vi "Panel Control State.vi"(8 "error in (no error)":errorcluster, 10 "Editable(True)":bool=TRUE, 11 "Panel Controls and VI Refnum":T1) -> (0 "error out":errorcluster, 3 "Panel Controls and VI Refnum out":T1)   [LabVIEW 2015, in "Panel Controller.lvclass"]
uses:
  Panel Controller.lvclass
  Panel Control/Panel Data/Type Definition/Panel Controls and VI Refnum.ctl
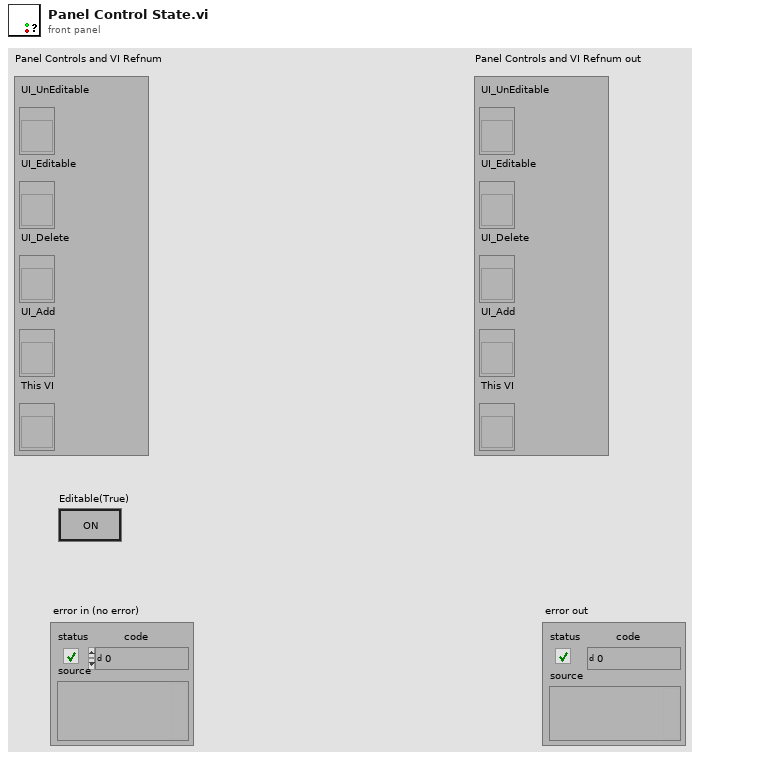
[diagram p1: front panel]
types:
  T1 = typedef "Panel Controller.lvclass/Panel Controls and VI Refnum.ctl" = cluster{"UI_UnEditable":refnum<vi>, "UI_Editable":refnum<vi>, "UI_Delete":refnum<vi>, "UI_Add":refnum<vi>, "This VI":refnum<vi>}
  T2 = enum8{"Enabled", "Disabled", "Disabled and Grayed Out"}
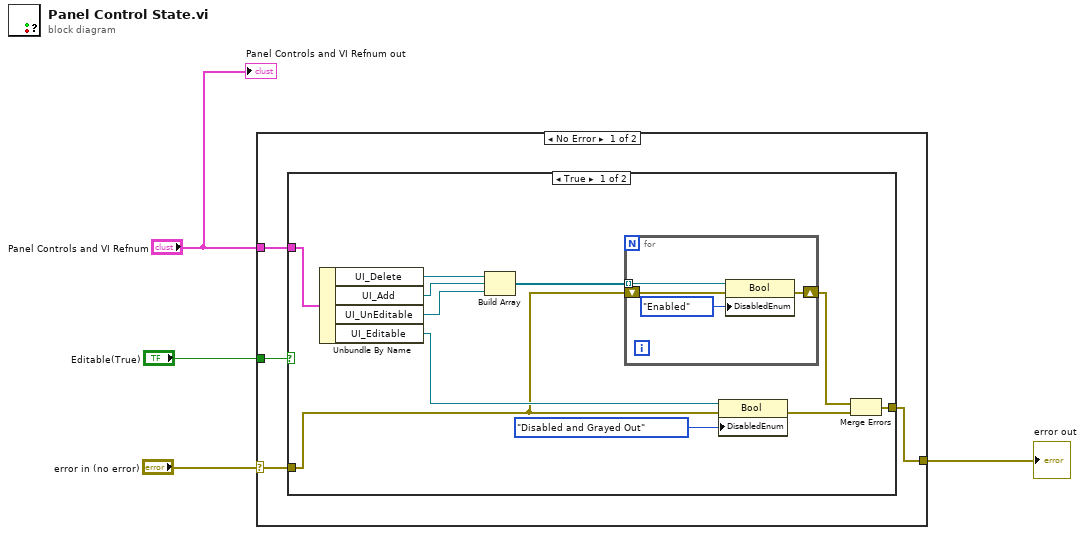
[diagram p0: block diagram]
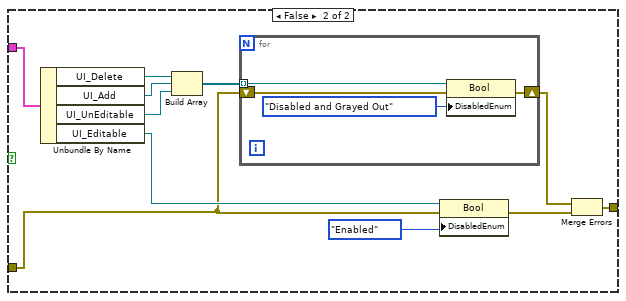
[diagram p2: hidden frame]
diagram:
  n1 = case shown="No Error" "error in (no error)" {
    selector: "error in (no error)" -> [w6 w39]
    tunnel: "Editable(True)" -> [w8 _]
    tunnel: "Panel Controls and VI Refnum" -> [w7 _]
    tunnel: [w5 w39] -> w1
    frame No Error {
      n2 = case shown="True" w8 {
        tunnel: w7 -> [w19 w34]
        tunnel: w6 -> [w12 w27]
        tunnel: [w9 w24] -> w5
        frame True {
          n3 = Unbundle By Name(w19) -> ("UI_Delete"=w18:refnum<vi>, "UI_Add"=w17:refnum<vi>, "UI_UnEditable"=w16:refnum<vi>, "UI_Editable"=w14:refnum<vi>)
          n4 = Build Array(w18, w17, w16) -> (w15:refnum<vi>[])
          n5 = for {
            tunnel: w15 -> [w23] mode=indexing
            shift-right: [w20] -> w11
            shift-left: w12 -> [w21]
            n6 = property class="Bool"(reference=w23, error in=w21, "DisabledEnum"=T2."Enabled" ("Disabled")) -> (error out=w20:errorcluster)  [unwired: 1 out]
          }
          n7 = property class="Bool"(reference=w14, error in=w12, "DisabledEnum"=T2."Disabled and Grayed Out" ("Disabled")) -> (error out=w10:errorcluster)  [unwired: 1 out]
          n8 = Merge Errors(w11, w10) -> (w9:errorcluster)
        }
        frame False {
          n9 = Unbundle By Name(w34) -> ("UI_Delete"=w33:refnum<vi>, "UI_Add"=w32:refnum<vi>, "UI_UnEditable"=w31:refnum<vi>, "UI_Editable"=w29:refnum<vi>)
          n10 = Build Array(w33, w32, w31) -> (w30:refnum<vi>[])
          n11 = for {
            tunnel: w30 -> [w38] mode=indexing
            shift-right: [w35] -> w26
            shift-left: w27 -> [w36]
            n12 = property class="Bool"(reference=w38, error in=w36, "DisabledEnum"=T2."Disabled and Grayed Out" ("Disabled")) -> (error out=w35:errorcluster)  [unwired: 1 out]
          }
          n13 = property class="Bool"(reference=w29, error in=w27, "DisabledEnum"=T2."Enabled" ("Disabled")) -> (error out=w25:errorcluster)  [unwired: 1 out]
          n14 = Merge Errors(w26, w25) -> (w24:errorcluster)
        }
      }
    }
    frame Error {
    }
  }
  "error out" <- w1
  "Panel Controls and VI Refnum out" <- "Panel Controls and VI Refnum"
